vi "EVM_Sweep_Only_LitePoint.vi"() -> ()   [LabVIEW 2023, in "EVM.lvlib"]
uses:
  lib/CTL/LitePoint_EVM_SG.ctl
  lib/CTL/LitePoint_EVM_SA.ctl
  EVM.lvlib
  lib/LitePoints/LitePoints.lvlib
  lib/FTDI/JIO/CLC_JIO_FTDI.lvlib
panel:
  out "Receoved Power":dbl format="%#.3g"
  out "error out":errorcluster
  in  "Power res":i32=2
  in  "Stop Power":i32=-10
  in  "Start Power":i32=-40
  in  "BFIC_ele_stop":i32=15
  in  "BFIC_ele_res":i32=3
  in  "BFIC_ele_start":i32
  in  "BFIC_com_stop":i32=15
  in  "BFIC_com_res":i32=3
  in  "BFIC_com_start":i32
  in  "UD_att_stop":i32=255
  in  "UD_att_res":i32=3
  in  "UD_att_start":i32
  out "UD_att":i32=45
  out "BFIC_com_step":i32=7
  out "BFIC_ele_step":i32=14
  out "SG Power":i32=-16
  in  "TRXmode":u16(ring)=1 items=["Tx"=1, "Rx"=2]
  in  "Polarity":u16(ring) items=["H", "V"]
  out "floder Exist?":bool=TRUE
  in  "Waiting \nTime(ms)":u32=1
  in  "FileNote":string="test4_wayne_MCS11"
  in  "SG":refnum<visa-resource-name>="IQXEL-M2X"
  in  "SA":refnum<visa-resource-name>="IQGIG"
  out "Spectrum Data":cluster{"X":dbl, "Y":dbl}[](graph)=[{"X"=-40.0, "Y"=-22.354872}, {"X"=-36.0, "Y"=-29.389366}, {"X"=-32.0, "Y"=-29.611685}, {"X"=-28.0, "Y"=-29.666927}, {"X"=-24.0, "Y"=-29.690155}, {"X"=-20.0, "Y"=-29.574627}]
  # "TMYTEK_CLC_JIO_LitePoint_EVM"
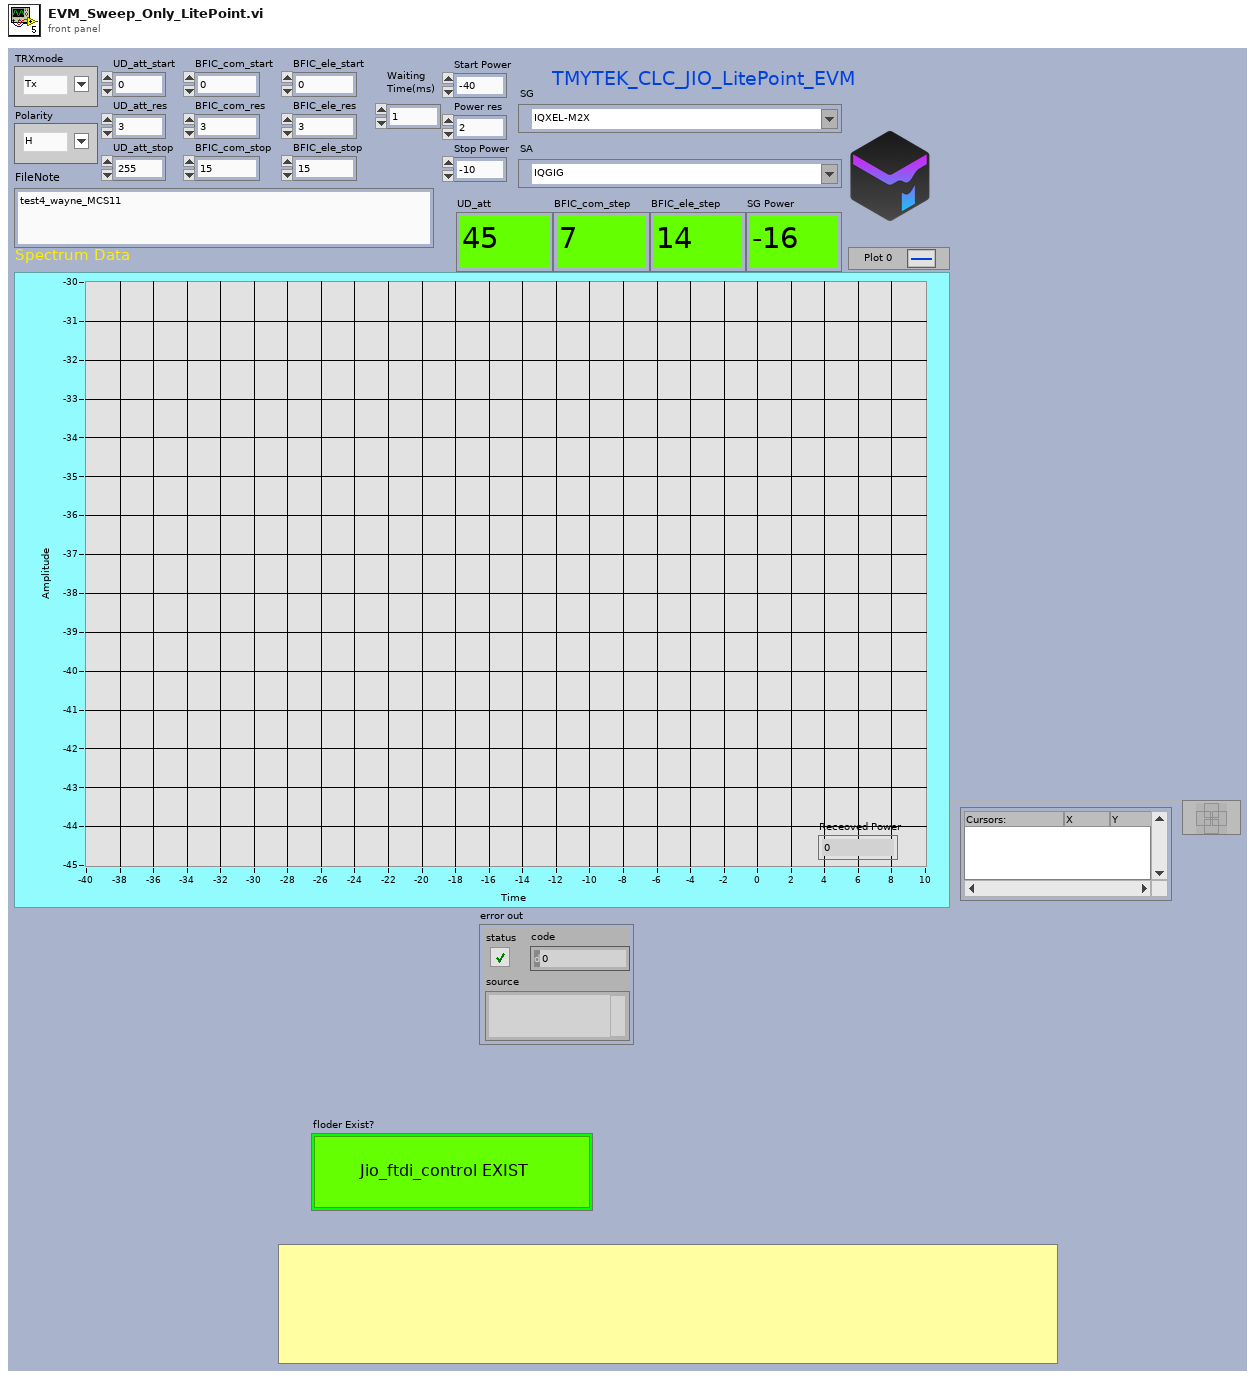
[diagram p1: front panel]
types:
  T1 = typedef "LitePoint_EVM_SG.ctl" = enum16{"Init", "Close", "set_SG", "AdjustLevel", "byPass", "RF_ON", "RF_OFF"}
  T2 = typedef "LitePoint_EVM_SA.ctl" = enum16{"Init", "Close", "set_SA", "get_EVM", "byPass", "getPower"}
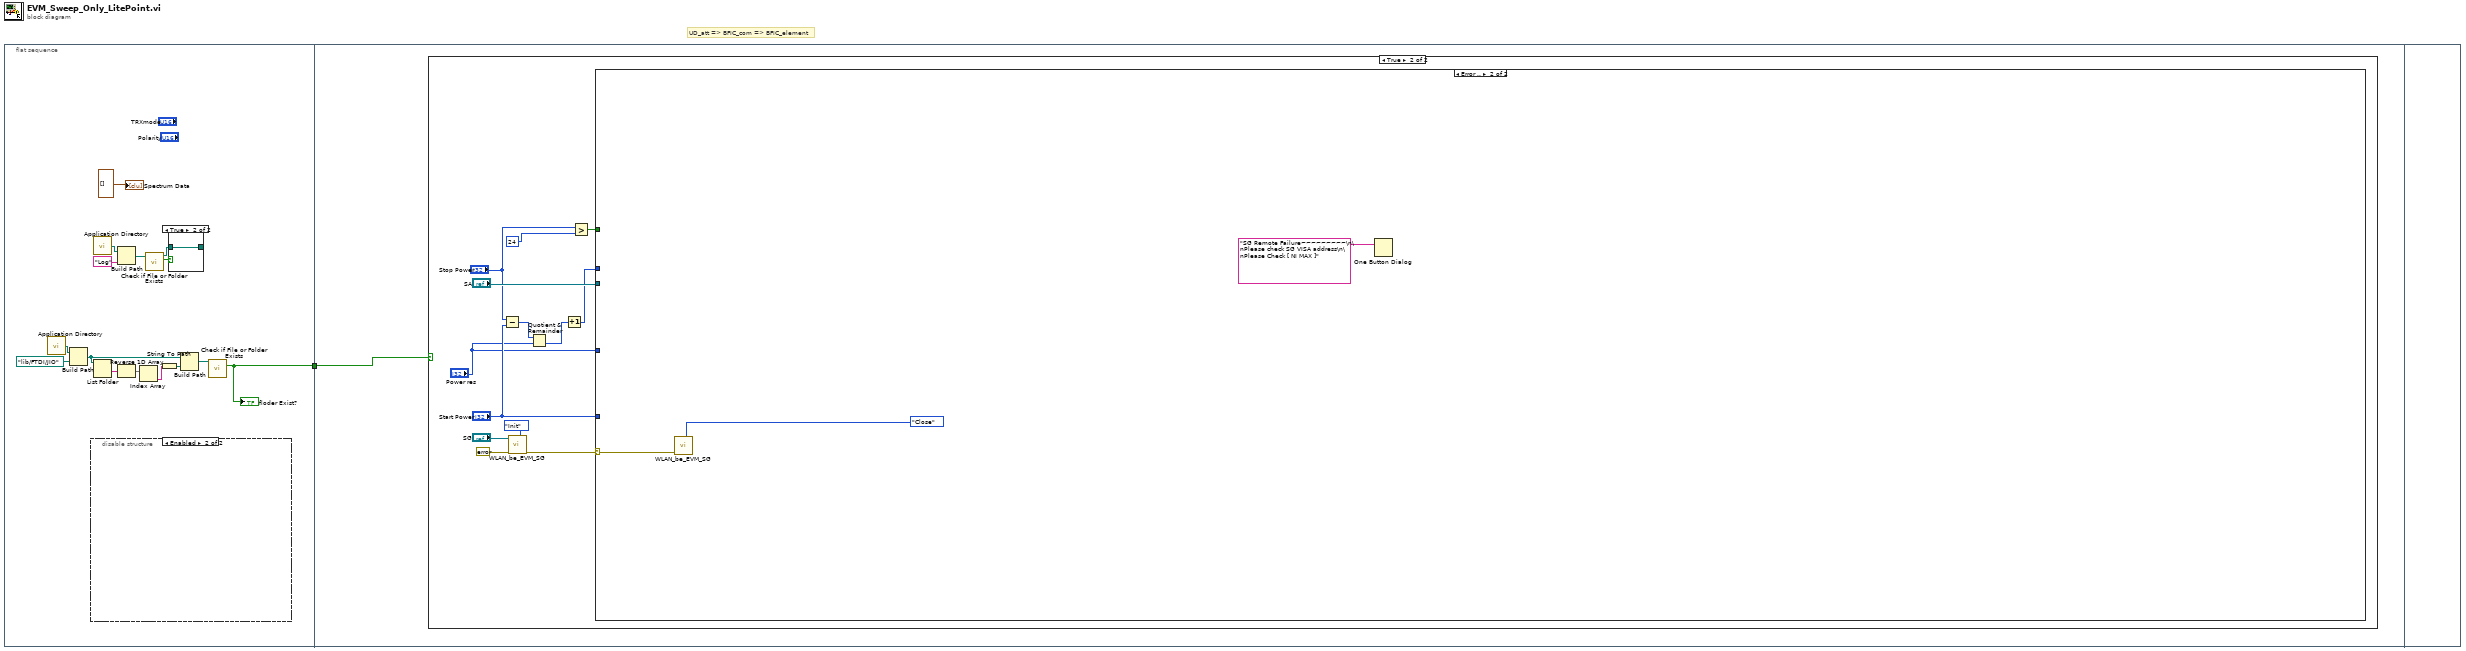
[diagram p0: block diagram]
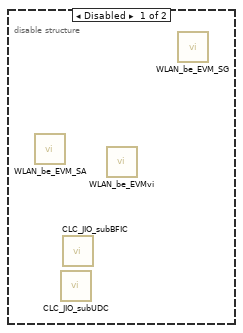
[diagram p2: hidden frame]
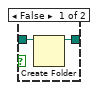
[diagram p3: hidden frame]
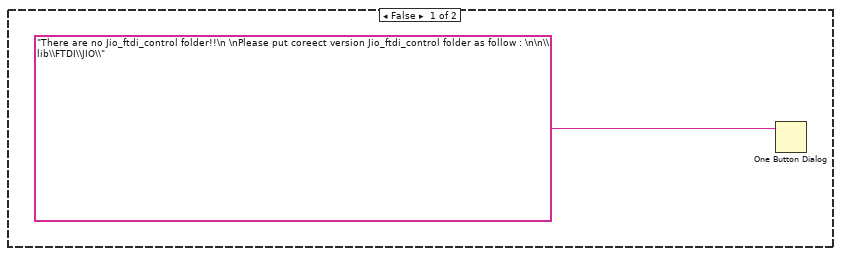
[diagram p4: hidden frame]
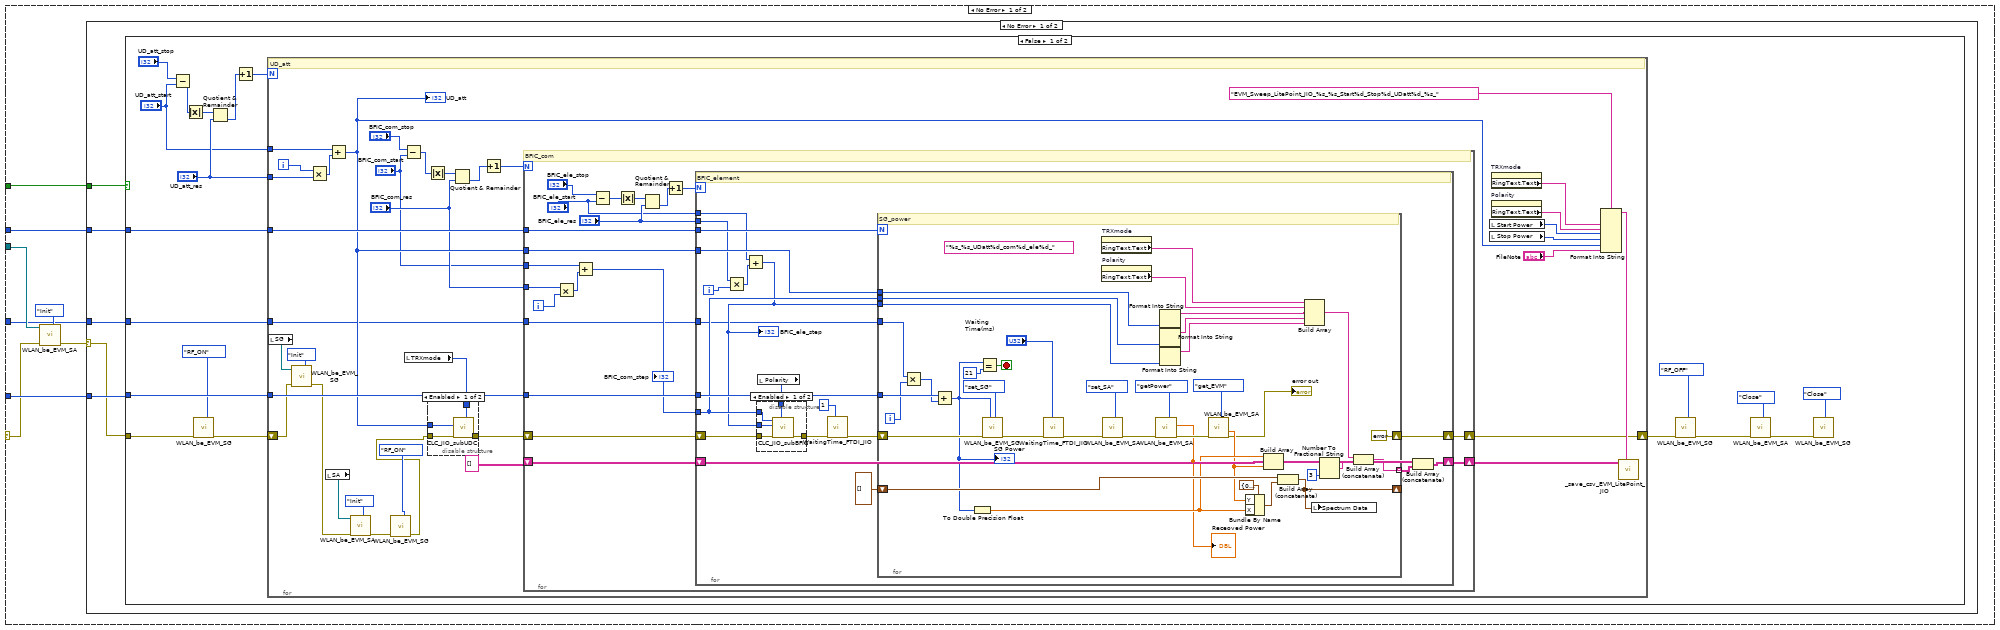
[diagram p5: hidden frame]
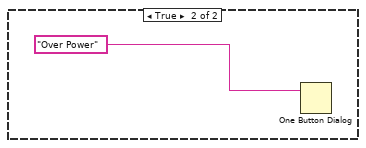
[diagram p8: hidden frame]
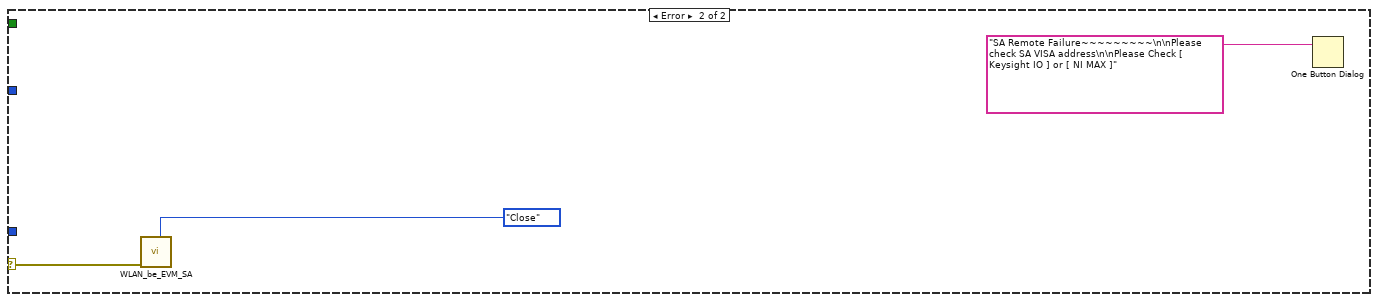
[diagram p9: hidden frame]
diagram:
  # "UD_att => BFIC_com => BFIC_element"
  n1 = flat-sequence {
    tunnel: [w2] -> w1
    tunnel: w1 -> [w20]
    frame #0 {
      n2 = call <vilib>:"Application Directory.vi"() -> ("Application Directory"=w8:path)
      n3 = Build Path(base path=w8, name or relative path=path "lib/FTDI/JIO") -> (appended path=w9:path)
      n4 = disable-structure shown="Enabled" {
        frame Disabled {
          n5 = call "WLAN_be_EVM_SA.vi"() -> ()  [unwired: 8 in, 4 out]
          n6 = call "CLC_JIO_subUDC.vi"() -> ()  [unwired: 10 in, 2 out]
          n7 = call "CLC_JIO_subBFIC.vi"() -> ()  [unwired: 10 in, 2 out]
          n8 = call "WLAN_be_EVMvi.vi"() -> ()  [unwired: 8 in, 4 out]
          n9 = call "WLAN_be_EVM_SG.vi"() -> ()  [unwired: 10 in, 2 out]
        }
        frame Enabled {
        }
      }
      n10 = call <vilib>:"Application Directory.vi"() -> ("Application Directory"=w15:path)
      n11 = List Folder(path=w9) -> (folder names=w4:string[])  [unwired: 3 in, 3 out]
      n12 = Reverse 1D Array(array=w4) -> (reversed array=w5:string[])
      n13 = Build Path(base path=w15, name or relative path="Log") -> (appended path=w12:path)
      n14 = Index Array(array=w5) -> (element=w6:string)  [unwired: 1 in]
      n15 = call <vilib>:"Check if File or Folder Exists.vi"("path"=w12) -> ("file or folder exists?"=w14:bool, "dup path"=w13:path)  [unwired: 8 in, 1 out]
      n16 = String To Path(string=w6) -> (path=w7:path)
      n17 = case shown="True" w14 {
        tunnel: w13 -> [w18 w19]
        tunnel: [w17 w19] -> _
        frame False {
          n18 = Create Folder(path (use dialog)=w18) -> (created path=w17:path)  [unwired: 2 in, 2 out]
        }
        frame True {
        }
      }
      n19 = Build Path(base path=w9, name or relative path=w7) -> (appended path=w10:path)
      n20 = call <vilib>:"Check if File or Folder Exists.vi"("path"=w10) -> ("file or folder exists?"=w2:bool)  [unwired: 8 in, 2 out]
      "floder Exist?" <- w2
      "Spectrum Data" <- cluster{"X":dbl, "Y":dbl}[] [] ("XY Graph")
    }
    frame #1 {
      n21 = case shown="True" w20 {
        frame False {
          n22 = One Button Dialog(message="There are no Jio_ftdi_control folder!!\n \nPlease put coreect version Jio_ftdi_control folder as follow : \n\n\\lib\\FTDI\\JIO\\") -> ()  [unwired: 1 in, 1 out]
        }
        frame True {
          n23 = Subtract(x="Stop Power", y="Start Power") -> (x-y=w24:i32)
          n24 = call "WLAN_be_EVM_SG.vi"("Function_SG"=LitePoint_EVM_SG."Init", "error in"=errorcluster {"status"=FALSE, "code"=0, "source"=""} ("error in (no error)"), "VISA IN"="SG") -> ("error out"=w27:errorcluster)  [unwired: 7 in, 1 out]
          n25 = Quotient & Remainder(x=w24, y="Power res") -> (floor(x/y)=w23:i32)  [unwired: 1 out]
          n26 = Increment(x=w23) -> (x+1=w31:i32)
          n27 = Greater?(x="Stop Power", y=24) -> (0:w33:bool)
          n28 = case shown="Error .." w27 {
            selector: w27 -> [w39 w198]
            tunnel: "SA" -> [w37 _]
            tunnel: w33 -> [w42 _]
            tunnel: "Start Power" -> [w41 _]
            tunnel: w31 -> [w40 _]
            tunnel: "Power res" -> [w35 _]
            frame No Error {
              n29 = call "WLAN_be_EVM_SA.vi"("Function"=LitePoint_EVM_SA."Init", "error in"=w39, "VISA IN"=w37) -> ("error out"=w38:errorcluster)  [unwired: 5 in, 3 out]
              n30 = case shown="No Error" w38 {
                selector: w38 -> [w44 w195]
                tunnel: w42 -> [w47 _]
                tunnel: w41 -> [w46 _]
                tunnel: w40 -> [w45 _]
                tunnel: w35 -> [w43 _]
                frame No Error {
                  n31 = case shown="False" w47 {
                    tunnel: w46 -> [w65 _]
                    tunnel: w44 -> [w64 _]
                    tunnel: w45 -> [w66 _]
                    tunnel: w43 -> [w48 _]
                    frame False {
                      n32 = Subtract(x="UD_att_stop", y="UD_att_start") -> (x-y=w55:i32)
                      n33 = Absolute Value(x=w55) -> (abs(x)=w52:i32)
                      n34 = call "WLAN_be_EVM_SG.vi"("Function_SG"=LitePoint_EVM_SG."RF_ON", "error in"=w64) -> ("error out"=w61:errorcluster)  [unwired: 8 in, 1 out]
                      n35 = Quotient & Remainder(x=w52, y="UD_att_res") -> (floor(x/y)=w53:i32)  [unwired: 1 out]
                      n36 = Increment(x=w53) -> (x+1=w49:i32)
                      n37 = for {
                        N: w49 -> [_]
                        tunnel: w66 -> [w102]
                        tunnel: w65 -> [w101]
                        shift-right: [w89] -> w60
                        shift-left: w61 -> [w74]
                        tunnel: "UD_att_res" -> [w86]
                        tunnel: "UD_att_start" -> [w85]
                        tunnel: w48 -> [w76]
                        i -> [w88]
                        # "UD_att"
                        n38 = local read "SG"() -> (w71:refnum<visa-resource-name>)
                        n39 = call "WLAN_be_EVM_SG.vi"("Function_SG"=LitePoint_EVM_SG."Init", "error in"=w74, "VISA IN"=w71) -> ("error out"=w72:errorcluster)  [unwired: 7 in, 1 out]
                        n40 = Multiply(x=w88, y=w86) -> (x*y=w87:i32)
                        n41 = local read "SA"() -> (w70:refnum<visa-resource-name>)
                        n42 = Add(x=w85, y=w87) -> (x+y=w84:i32)
                        "UD_att" <- w84
                        n43 = call "WLAN_be_EVM_SA.vi"("Function"=LitePoint_EVM_SA."Init", "error in"=w72, "VISA IN"=w70) -> ("error out"=w68:errorcluster)  [unwired: 5 in, 3 out]
                        n44 = call "WLAN_be_EVM_SG.vi"("Function_SG"=LitePoint_EVM_SG."RF_ON", "error in"=w68) -> ("error out"=w67:errorcluster)  [unwired: 8 in, 1 out]
                        n45 = Subtract(x="BFIC_com_stop", y="BFIC_com_start") -> (x-y=w83:i32)
                        n46 = local read "TRXmode"() -> (w98:u16)
                        n47 = disable-structure shown="Enabled" {
                          disable-tunnel: [w106 w107] -> w100
                          disable-tunnel: w67 -> [w105 w107]
                          disable-tunnel: w98 -> [w104 _]
                          disable-tunnel: w84 -> [w103 _]
                          frame Enabled {
                            n48 = call "CLC_JIO_subUDC.vi"("Mode"=w104, "error in"=w105, "ud att"=w103) -> ("error out"=w106:errorcluster)  [unwired: 7 in, 1 out]
                          }
                          frame Disabled {
                          }
                        }
                        n49 = Absolute Value(x=w83) -> (abs(x)=w82:i32)
                        n50 = Quotient & Remainder(x=w82, y="BFIC_com_res") -> (floor(x/y)=w78:i32)  [unwired: 1 out]
                        n51 = Increment(x=w78) -> (x+1=w77:i32)
                        n52 = for {
                          N: w77 -> [_]
                          tunnel: w102 -> [w127]
                          tunnel: w101 -> [w126]
                          shift-right: [w123] -> w99
                          shift-left: string[][] [] -> [w124]
                          tunnel: w84 -> [w122]
                          shift-right: [w121] -> w89
                          shift-left: w100 -> [w125]
                          tunnel: "BFIC_com_res" -> [w117]
                          tunnel: "BFIC_com_start" -> [w116]
                          tunnel: w76 -> [w108]
                          i -> [w119]
                          # "BFIC_com"
                          n53 = Multiply(x=w117, y=w119) -> (x*y=w120:i32)
                          n54 = Add(x=w116, y=w120) -> (x+y=w118:i32)
                          "BFIC_com_step" <- w118
                          n55 = Subtract(x="BFIC_ele_stop", y="BFIC_ele_start") -> (x-y=w114:i32)
                          n56 = Absolute Value(x=w114) -> (abs(x)=w115:i32)
                          n57 = Quotient & Remainder(x=w115, y="BFIC_ele_res") -> (floor(x/y)=w112:i32)  [unwired: 1 out]
                          n58 = Increment(x=w112) -> (x+1=w109:i32)
                          n59 = for {
                            N: w109 -> [_]
                            tunnel: w127 -> [w147]
                            tunnel: w126 -> [w145]
                            shift-right: [w143] -> w123
                            shift-left: w124 -> [w142]
                            tunnel: w118 -> [w136]
                            tunnel: w122 -> [w137]
                            shift-right: [w134] -> w121
                            shift-left: w125 -> [w141]
                            tunnel: "BFIC_ele_res" -> [w130]
                            tunnel: "BFIC_ele_start" -> [w129]
                            tunnel: w108 -> [w128]
                            i -> [w131]
                            # "BFIC_element"
                            n60 = Multiply(x=w130, y=w131) -> (x*y=w133:i32)
                            n61 = Add(x=w129, y=w133) -> (x+y=w132:i32)
                            "BFIC_ele_step" <- w132
                            n62 = local read "Polarity"() -> (w135:u16)
                            n63 = disable-structure shown="Enabled" {
                              disable-tunnel: w141 -> [w152 w153]
                              disable-tunnel: [w151 w153] -> w140
                              disable-tunnel: w132 -> [w150 _]
                              disable-tunnel: w136 -> [w149 _]
                              disable-tunnel: w135 -> [w148 _]
                              frame Enabled {
                                n64 = call "CLC_JIO_subBFIC.vi"("pol"=w148, "error in"=w152, "ele"=w150, "com"=w149) -> ("error out"=w151:errorcluster)  [unwired: 6 in, 1 out]
                              }
                              frame Disabled {
                              }
                            }
                            n65 = call "WaitingTime_FTDI_JIO.vi"("Waiting Time(ms)"=u32 1, "error out"=w140) -> ("error out"=w139:errorcluster)  [unwired: 9 in]
                            n66 = for {
                              N: w147 -> [_]
                              tunnel: w145 -> [w192]
                              shift-right: [errorcluster {"status"=FALSE, "code"=0, "source"=""} ("error out")] -> w134
                              shift-left: w139 -> [w184]
                              shift-right: [w186] -> _
                              shift-left: cluster{"X":dbl, "Y":dbl}[] [] ("XY Graph") -> [w188]
                              tunnel: [w168] -> w144 mode=indexing
                              tunnel: w137 -> [w165]
                              tunnel: w132 -> [w163]
                              tunnel: w136 -> [w164]
                              tunnel: w128 -> [w157]
                              i -> [w158]
                              stop <- w190 stop-if-true
                              (unwired) "%s_%s_UDatt%d_com%d_ele%d_" ("format string")
                              # "SG_power"
                              n67 = Multiply(x=w157, y=w158) -> (x*y=w156:i32)
                              n68 = Add(x=w192, y=w156) -> (x+y=w183:i32)
                              "SG Power" <- w183
                              n69 = To Double Precision Float(number=w183) -> (double precision float=w185:dbl)
                              n70 = Equal?(x=w183, y=21) -> (x = y?=w190:bool)
                              n71 = call "WLAN_be_EVM_SG.vi"("Function_SG"=LitePoint_EVM_SG."set_SG", "setPower"=w183, "error in"=w184) -> ("error out"=w174:errorcluster)  [unwired: 7 in, 1 out]
                              n72 = call "WaitingTime_FTDI_JIO.vi"("Waiting Time(ms)"="Waiting \nTime(ms)", "error out"=w174) -> ("error out"=w173:errorcluster)  [unwired: 9 in]
                              n73 = property on="TRXmode" class="Ring (strict)"() -> ("RingText.Text"=w167:string)  [unwired: 2 in, 2 out]
                              n74 = property on="Polarity" class="Ring (strict)"() -> ("RingText.Text"=w166:string)  [unwired: 2 in, 2 out]
                              n75 = call "WLAN_be_EVM_SA.vi"("Function"=LitePoint_EVM_SA."set_SA", "error in"=w173) -> ("error out"=w180:errorcluster)  [unwired: 6 in, 3 out]
                              n76 = call "WLAN_be_EVM_SA.vi"("Function"=LitePoint_EVM_SA."getPower", "error in"=w180) -> ("error out"=w178:errorcluster, "Power"=w176:dbl)  [unwired: 6 in, 2 out]
                              "Receoved Power" <- w176
                              n77 = Format Into String(w165) -> (resulting string=w162:string)  [unwired: 3 in, 1 out]
                              n78 = Format Into String(w164) -> (resulting string=w161:string)  [unwired: 3 in, 1 out]
                              n79 = Format Into String(w163) -> (resulting string=w160:string)  [unwired: 3 in, 1 out]
                              n80 = call "WLAN_be_EVM_SA.vi"("Function"=LitePoint_EVM_SA."get_EVM", "error in"=w178) -> ("error out"=→"error out":errorcluster, "EVM"=w175:dbl)  [unwired: 6 in, 2 out]
                              n81 = Bundle By Name(cluster=cluster{"X":dbl, "Y":dbl} {"X"=0.0, "Y"=0.0} ("element"), "Y"=w175, "X"=w185) -> (w187:cluster{"X":dbl, "Y":dbl})
                              n82 = Build Array(w185, w176, w175) -> (w170:dbl[])
                              n83 = Build Array (concatenate)(w188, w187) -> (w186:cluster{"X":dbl, "Y":dbl}[])
                              n84 = Build Array(w167, w166, w162, w161, w160) -> (w159:string[])
                              n85 = local write "Spectrum Data"(w186) -> ()
                              n86 = Number To Fractional String(number=w170, precision (6)=i16 3) -> (F-format string=w169:string[])  [unwired: 2 in]
                              n87 = Build Array (concatenate)(w159, w169) -> (w168:string[])
                            }
                            n88 = Build Array (concatenate)(w142, w144) -> (w143:string[][])
                          }
                        }
                        n89 = local read "Start Power"() -> (w93:i32)
                        n90 = local read "Stop Power"() -> (w95:i32)
                        n91 = property on="TRXmode" class="Ring (strict)"() -> ("RingText.Text"=w91:string)  [unwired: 2 in, 2 out]
                        n92 = property on="Polarity" class="Ring (strict)"() -> ("RingText.Text"=w92:string)  [unwired: 2 in, 2 out]
                        n93 = Format Into String(format string="EVM_Sweep_LitePoint_JIO_%s_%s_Start%d_Stop%d_UDatt%d_%s_" ("delimiter (\\t)"), w91, w92, w93, w95, w84, "FileNote") -> (resulting string=w96:string)  [unwired: 2 in, 1 out]
                        n94 = call "_save_csv_EVM_LitePoint_JIO.vi"("delimiter (\\t)"=w96, "array in"=w99) -> ()  [unwired: 9 in, 1 out]
                      }
                      n95 = call "WLAN_be_EVM_SG.vi"("Function_SG"=LitePoint_EVM_SG."RF_OFF", "error in"=w60) -> ("error out"=w57:errorcluster)  [unwired: 8 in, 1 out]
                      n96 = call "WLAN_be_EVM_SA.vi"("Function"=LitePoint_EVM_SA."Close", "error in"=w57) -> ("error out"=w56:errorcluster)  [unwired: 6 in, 3 out]
                      n97 = call "WLAN_be_EVM_SG.vi"("Function_SG"=LitePoint_EVM_SG."Close", "error in"=w56) -> ()  [unwired: 8 in, 2 out]
                    }
                    frame True {
                      n98 = One Button Dialog(message="Over Power") -> ()  [unwired: 1 in, 1 out]
                    }
                  }
                }
                frame Error {
                  n99 = call "WLAN_be_EVM_SA.vi"("Function"=LitePoint_EVM_SA."Close", "error in"=w195) -> ()  [unwired: 6 in, 4 out]
                  n100 = One Button Dialog(message="SA Remote Failure~~~~~~~~~\n\nPlease check SA VISA address\n\nPlease Check [ Keysight IO ] or [ NI MAX ]") -> ()  [unwired: 1 in, 1 out]
                }
              }
            }
            frame Error {
              n101 = call "WLAN_be_EVM_SG.vi"("Function_SG"=LitePoint_EVM_SG."Close", "error in"=w198) -> ()  [unwired: 8 in, 2 out]
              n102 = One Button Dialog(message="SG Remote Failure~~~~~~~~~\n\nPlease check SG VISA address\n\nPlease Check [ NI MAX ]") -> ()  [unwired: 1 in, 1 out]
            }
          }
        }
      }
    }
    frame #2 {
    }
  }
